vi "NXT SendData.vi"(6 "error in (no error)":errorcluster, 8 "Data":u8[](array[numeric])) -> (0 "error out":errorcluster)   [LabVIEW 2012]
uses:
  <vilib>/NXT/NXT Controls/NXTSyscallRefnum.ctl
  <resource>/objmgr/NXTInputOutput.rc
panel:
  in  "Sys Call Refnum":T1
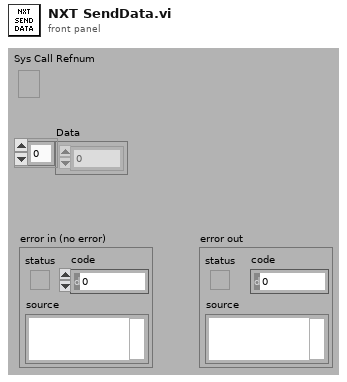
[diagram p1: front panel]
types:
  T1 = typedef "NXTSyscallRefnum.ctl" = refnum<k21>
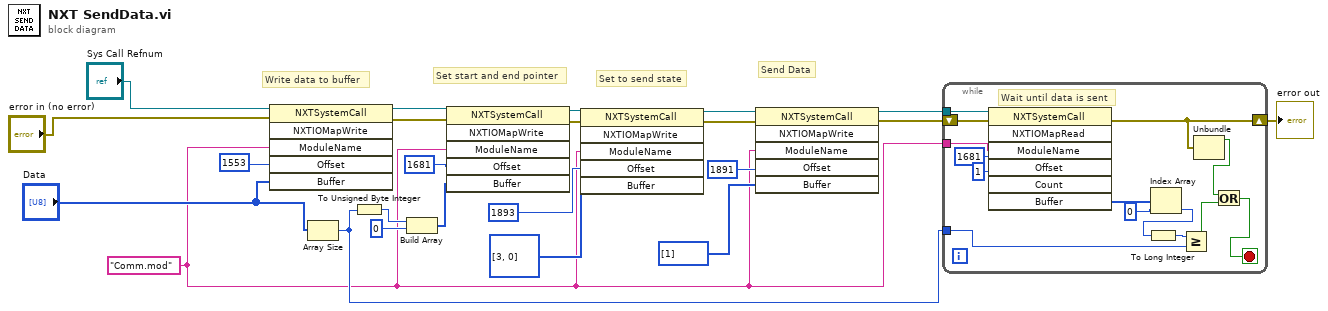
[diagram p0: block diagram]
diagram:
  w1 = "Comm.mod" ("ModuleName")
  # "Send Data"
  # "Set to send state"
  # "Set start and end pointer"
  # "Write data to buffer"
  n1 = invoke class="NXTSystemCall" method="NXTIOMapWrite"(reference="Sys Call Refnum", error in="error in (no error)", "ModuleName"=w1, "Offset"=u16 1553, "Buffer"="Data") -> (reference out=w22:T1, error out=w21:errorcluster)  [unwired: 1 in, 4 out]
  n2 = Array Size(array="Data") -> (size(s)=w2:i32)
  n3 = To Unsigned Byte Integer(number=w2) -> (unsigned 8bit integer=w3:u8)
  n4 = Build Array(w3, u8 0 ("element")) -> (w9:u8[])
  n5 = invoke class="NXTSystemCall" method="NXTIOMapWrite"(reference=w22, error in=w21, "ModuleName"=w1, "Offset"=u16 1681, "Buffer"=w9) -> (reference out=w19:T1, error out=w18:errorcluster)  [unwired: 1 in, 4 out]
  n6 = invoke class="NXTSystemCall" method="NXTIOMapWrite"(reference=w19, error in=w18, "ModuleName"=w1, "Offset"=u16 1893, "Buffer"=u8[] [3, 0]) -> (reference out=w12:T1, error out=w13:errorcluster)  [unwired: 1 in, 4 out]
  n7 = invoke class="NXTSystemCall" method="NXTIOMapWrite"(reference=w12, error in=w13, "ModuleName"=w1, "Offset"=u16 1891, "Buffer"=u8[] [1]) -> (reference out=w7:T1, error out=w6:errorcluster)  [unwired: 1 in, 4 out]
  n8 = while {
    tunnel: w7 -> [w33]
    tunnel: w1 -> [w31]
    tunnel: w2 -> [w30]
    shift-right: [w29] -> w5
    shift-left: w6 -> [w32]
    stop <- w24 stop-if-true
    # "Wait until data is sent"
    n9 = invoke class="NXTSystemCall" method="NXTIOMapRead"(reference=w33, error in=w32, "ModuleName"=w31, "Offset"=u16 1681, "Count"=u16 1) -> (error out=w29:errorcluster, "Buffer"=w35:u8[])  [unwired: 2 in, 5 out]
    n10 = Index Array(array=w35, index=0) -> (element=w26:u8)
    n11 = To Long Integer(number=w26) -> (32bit integer=w25:i32)
    n12 = Greater Or Equal?(x=w25, y=w30) -> (x >= y?=w28:bool)
    n13 = Unbundle(w29) -> ("status"=w27:bool)  [unwired: 2 out]
    n14 = Or(x=w27, y=w28) -> (x .or. y?=w24:bool)
  }
  "error out" <- w5
